vi "assemble images.vi"(6 "bidi_y":bool, 7 "bidi_x":bool, 8 "y pixels":i32=200 min=2 max=1024 step=1, 9 "bin factor":dbl, 10 "x pixels":i32=200 min=2 max=1024 step=1, 11 "raw data in (negative 11 bit data)":i16[](array[numeric])) -> (2 "second image":dbl[][](array[numeric]), 3 "first image":dbl[][](array[numeric]))   [LabVIEW 2012]
doc: "SciScan 1.2 160622"
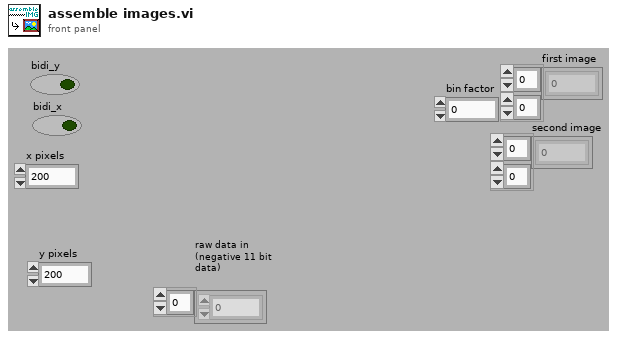
[diagram p1: front panel]
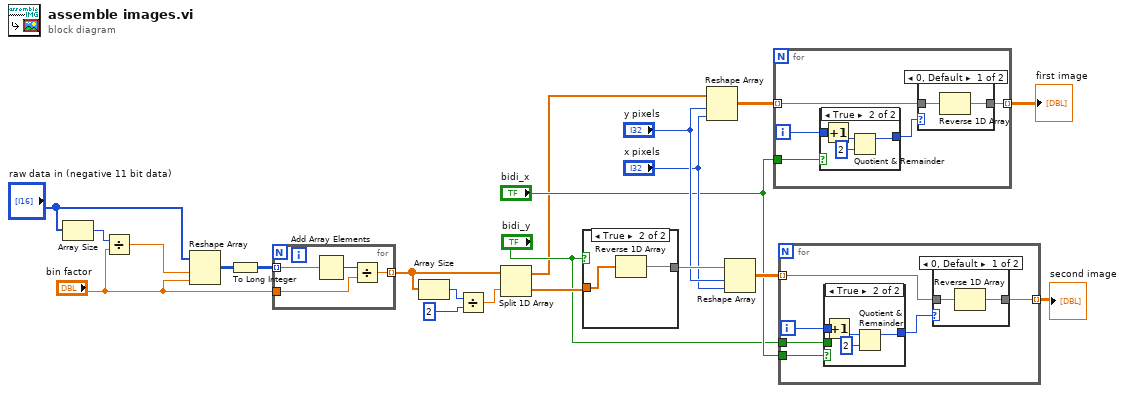
[diagram p0: block diagram]
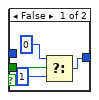
[diagram p3: hidden frame]
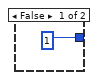
[diagram p5: hidden frame]
diagram:
  n1 = Array Size(array="raw data in (negative 11 bit data)") -> (size(s)=w7:i32)
  n2 = Divide(x=w7, y="bin factor") -> (x/y=w21:dbl)
  n3 = Reshape Array("raw data in (negative 11 bit data)", w21, "bin factor") -> (w20:i16[][])
  n4 = To Long Integer(number=w20) -> (32bit integer=w19:i32[][])
  n5 = for {
    tunnel: w19 -> [w24] mode=indexing
    tunnel: [w23] -> w14 mode=indexing
    tunnel: "bin factor" -> [w22]
    n6 = Add Array Elements(numeric array=w24) -> (sum=w25:i32)
    n7 = Divide(x=w25, y=w22) -> (x/y=w23:dbl)
  }
  n8 = Array Size(array=w14) -> (size(s)=w18:i32)
  n9 = Divide(x=w18, y=2) -> (x/y=w11:dbl)
  n10 = Split 1D Array(array=w14, index=w11) -> (first subarray=w1:dbl[], second subarray=w16:dbl[])
  n11 = case shown="True" "bidi_y" {
    tunnel: w16 -> [w26 w28]
    tunnel: [w26 w27] -> w15
    frame False {
    }
    frame True {
      n12 = Reverse 1D Array(array=w28) -> (reversed array=w27:dbl[])
    }
  }
  n13 = Reshape Array(w1, "y pixels", "x pixels") -> (w13:dbl[][])
  n14 = Reshape Array(w15, "y pixels", "x pixels") -> (w4:dbl[][])
  n15 = for {
    tunnel: w13 -> [w31] mode=indexing
    tunnel: [w30] -> w12 mode=indexing
    tunnel: "bidi_x" -> [w29]
    i -> [w33]
    n16 = case shown="True" w29 {
      tunnel: w33 -> [_ w38]
      tunnel: [1 w36] -> w32
      frame False {
      }
      frame True {
        n17 = Increment(x=w38) -> (x+1=w35:i32)
        n18 = Quotient & Remainder(x=w35, y=2) -> (x-y*floor(x/y)=w36:i32)  [unwired: 1 out]
      }
    }
    n19 = case shown="0, Default" w32 {
      tunnel: w31 -> [w40 w41]
      tunnel: [w39 w41] -> w30
      frame 0, Default {
        n20 = Reverse 1D Array(array=w40) -> (reversed array=w39:dbl[])
      }
      frame 1 {
      }
    }
  }
  "first image" <- w12
  n21 = for {
    tunnel: w4 -> [w45] mode=indexing
    tunnel: [w44] -> w5 mode=indexing
    tunnel: "bidi_x" -> [w43]
    tunnel: "bidi_y" -> [w42]
    i -> [w47]
    n22 = case shown="True" w43 {
      tunnel: w47 -> [_ w58]
      tunnel: [w52 w56] -> w46
      tunnel: w42 -> [w53 _]
      frame False {
        n23 = Select(t=0, s=w53, f=1) -> (s? t:f=w52:i32)
      }
      frame True {
        n24 = Increment(x=w58) -> (x+1=w55:i32)
        n25 = Quotient & Remainder(x=w55, y=2) -> (x-y*floor(x/y)=w56:i32)  [unwired: 1 out]
      }
    }
    n26 = case shown="0, Default" w46 {
      tunnel: w45 -> [w49 w50]
      tunnel: [w48 w50] -> w44
      frame 0, Default {
        n27 = Reverse 1D Array(array=w49) -> (reversed array=w48:dbl[])
      }
      frame 1 {
      }
    }
  }
  "second image" <- w5
